vi "DACSinglePoint.vi"() -> ()   [LabVIEW 2021]
uses:
  <vilib>/Utility/error.llb/DialogType.ctl
  <vilib>/DAQmx/write.llb/DAQmx Write (Analog 1D DBL NChan 1Samp).vi
  <vilib>/DAQmx/miscellaneous.llb/DAQmx Fill In Error Info.vi
  <vilib>/DAQmx/create/channels.llb/DAQmx Create Channel (AO-Voltage-Basic).vi
  <resource>/objmgr/daqmx.rc
panel:
  in  "Values":T1(array[cluster]) {"Coef" format="%#_3g"; "Value" format="%#_3p"}
  out "message":string
  out "Error":bool
  out "NumChans":u32
  in  "Enable":bool
  in  "Physical channels":tag
  # "(Label, Value, Coefficient)"
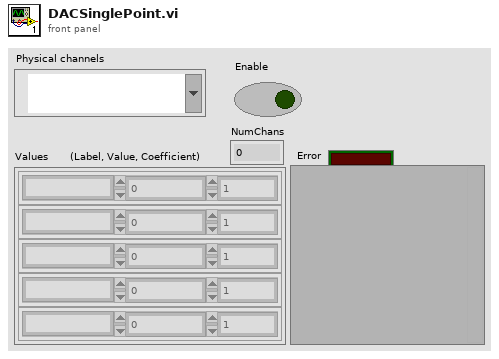
[diagram p1: front panel]
types:
  T1 = cluster{"Name":string, "Value":dbl, "Coef":dbl}[]
  T2 = typedef "DialogType.ctl" = u16
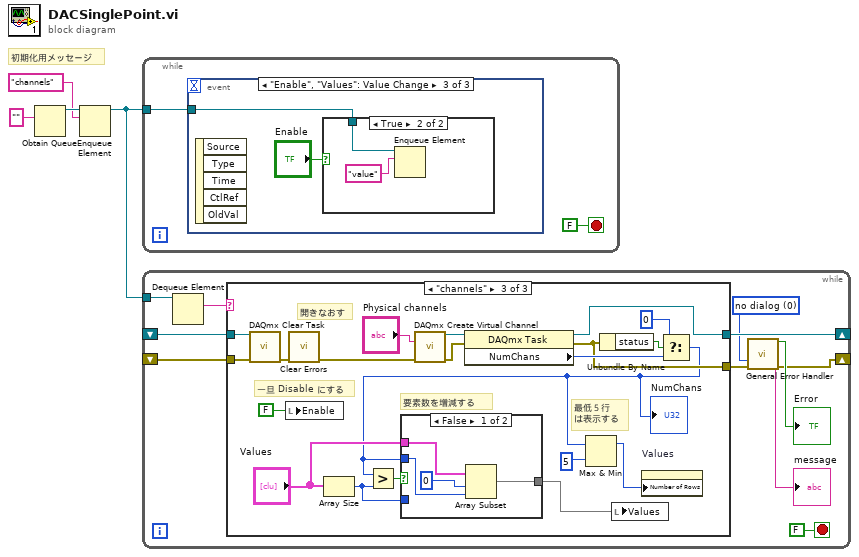
[diagram p0: block diagram]
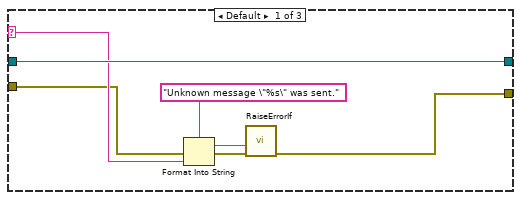
[diagram p2: hidden frame]
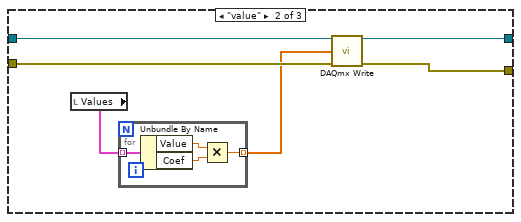
[diagram p3: hidden frame]
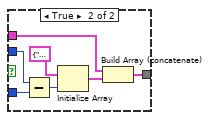
[diagram p4: hidden frame]
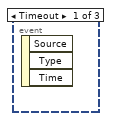
[diagram p5: hidden frame]
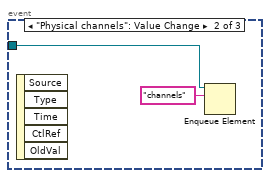
[diagram p6: hidden frame]
diagram:
  # "初期化用メッセージ"
  n1 = Obtain Queue(element data type="") -> (queue out=w3:refnum<queue>)  [unwired: 4 in, 2 out]
  n2 = Enqueue Element(queue=w3, element="channels") -> (queue out=w1:refnum<queue>)  [unwired: 2 in, 2 out]
  n3 = while {
    tunnel: w1 -> [w5]
    stop <- FALSE stop-if-true
    n4 = event shown="[2] \"Enable\", \"Values\": Value Change" {
      selector: _ -> [_ _ _]
      dyn-events: _ -> [_ _ _]
      timeout: _ -> [_ _ _]
      tunnel: w5 -> [_ w8 w10]
      event Timeout {
        n5 = event-data() -> ()  [unwired: 1 in, 3 out]
      }
      event "Physical channels": Value Change {
        n6 = event-data() -> ()  [unwired: 1 in, 5 out]
        n7 = Enqueue Element(queue=w8, element="channels") -> ()  [unwired: 2 in, 3 out]
      }
      event "Enable", "Values": Value Change {
        n8 = event-data() -> ()  [unwired: 1 in, 5 out]
        n9 = case shown="True" "Enable" {
          tunnel: w10 -> [_ w12]
          frame False {
          }
          frame True {
            n10 = Enqueue Element(queue=w12, element="value") -> ()  [unwired: 2 in, 3 out]
          }
        }
      }
    }
  }
  n11 = while {
    tunnel: w1 -> [w23]
    shift-right: [w20] -> _
    shift-left: _ -> [w19]
    shift-right: [w14] -> _
    shift-left: _ -> [w18]
    stop <- FALSE stop-if-true
    w13 = T2 0 items=["no dialog", "OK message", "continue or stop message", "OK message + warnings", "continue/stop + warnings"] ("type of dialog (OK msg:1)")
    n12 = Dequeue Element(queue=w23) -> (element=w21:string)  [unwired: 2 in, 3 out]
    n13 = case shown="\"channels\"" w21 {
      selector: w21 -> [w29 _ _]
      tunnel: [w30 w35 w57] -> w20
      tunnel: w19 -> [w30 w36 w56]
      tunnel: [w25 w33 w50] -> w17
      tunnel: w18 -> [w27 w34 w54]
      frame Default {
        n14 = Format Into String(format string="Unknown message \"%s\" was sent.", error in=w27, w29) -> (resulting string=w24:string, error out=w26:errorcluster)  [unwired: 1 in]
        n15 = call "RaiseErrorIf.vi"("error in (no error)"=w26, "error message"=w24) -> ("error out"=w25:errorcluster)  [unwired: 9 in]
      }
      frame "value" {
        n16 = local read "Values"() -> (w31:T1)
        n17 = for {
          tunnel: [w37] -> w32 mode=indexing
          tunnel: w31 -> [w40] mode=indexing
          n18 = Unbundle By Name(w40) -> ("Value"=w38:dbl, "Coef"=w39:dbl)
          n19 = Multiply(x=w38, y=w39) -> (x*y=w37:dbl)
        }
        n20 = call-poly <vilib>:"DAQmx Write.vi"("task/channels in"=w36, "data"=w32, "error in"=w34) -> ("task out"=w35:refnum<k21>, "error out"=w33:errorcluster)  [unwired: 10 in, 1 out]
      }
      frame "channels" {
        # "最低５行\nは表示する"
        # "開きなおす"
        # "要素数を増減する"
        # "一旦 Disable にする"
        n21 = call <vilib>:"DAQmx Clear Task.vi"("task in"=w56, "error in"=w54) -> ("error out"=w49:errorcluster)  [unwired: 13 in]
        n22 = local write "Enable"(FALSE ("Enable")) -> ()
        n23 = call <vilib>:"Clear Errors.vi"("error in (no error)"=w49) -> ("error out"=w48:errorcluster)  [unwired: 5 in, 1 out]
        n24 = Array Size(array="Values") -> (size(s)=w45:i32)
        n25 = call-poly <vilib>:"DAQmx Create Virtual Channel.vi"("physical channels"="Physical channels", "error in"=w48) -> ("task out"=w59:refnum<k21>, "error out"=w60:errorcluster)  [unwired: 12 in]
        n26 = property class="DAQmx Task"(reference=w59, error in=w60) -> (reference out=w57:refnum<k21>, error out=w50:errorcluster, "NumChans"=w52:u32)
        n27 = Unbundle By Name(w50) -> ("status"=w53:bool)
        n28 = Select(t=u32 0, s=w53, f=w52) -> (s? t:f=w42:u32)
        "NumChans" <- w42
        n29 = Greater?(x=w42, y=w45) -> (0:w47:bool)
        n30 = case shown="False" w47 {
          tunnel: "Values" -> [w64 w66]
          tunnel: w42 -> [w61 w71]
          tunnel: w45 -> [_ w70]
          tunnel: [w62 w68] -> w44
          frame False {
            n31 = Array Subset(array=w64, index=0, length=w61) -> (w62:T1)
          }
          frame True {
            n32 = Subtract(x=w71, y=w70) -> (x-y=w69:u32)
            n33 = Initialize Array(cluster{"Name":string, "Value":dbl, "Coef":dbl} {"Name"="", "Value"=0.0, "Coef"=1.0} ("Cluster"), w69) -> (w67:T1)
            n34 = Build Array (concatenate)(w66, w67) -> (w68:T1)
          }
        }
        n35 = Max & Min(x=w42, y=u32 5 ("s? t:f")) -> (max(x,y)=w41:u32)  [unwired: 1 out]
        n36 = local write "Values"(w44) -> ()
        n37 = property on="Values" class="Arr (strict)"("Number of Rows"=w41) -> ()  [unwired: 2 in, 2 out]
      }
    }
    n38 = call <vilib>:"General Error Handler.vi"("type of dialog (OK msg:1)"=w13, "error in (no error)"=w17) -> ("error?"=→"Error":bool, "message"=→"message":string, "error out"=w14:errorcluster)  [unwired: 9 in, 2 out]
  }
